vi "LTESaveDataReal1.vi"(7 "Boolean":bool, 8 "error in":errorcluster, 9 "varName":string, 10 "real1":dbl[](array[numeric])=[1.0, 2.0, 3.0], 11 "Path":path=path "C:/Users/Administrator/Desktop") -> (0 "error IO":errorcluster)   [LabVIEW 2015]
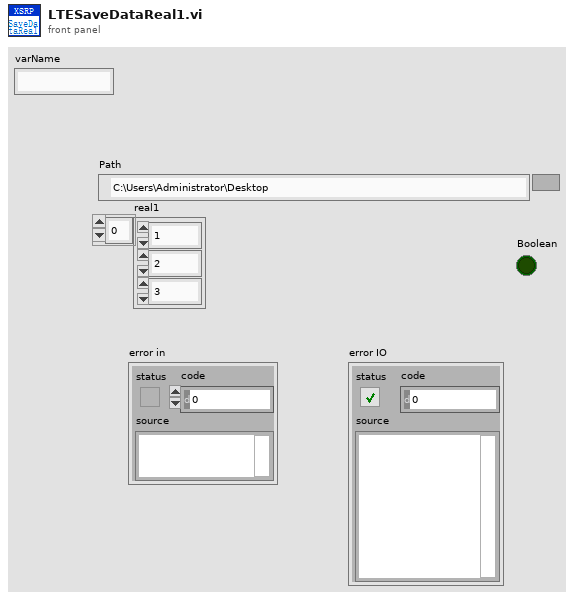
[diagram p1: front panel]
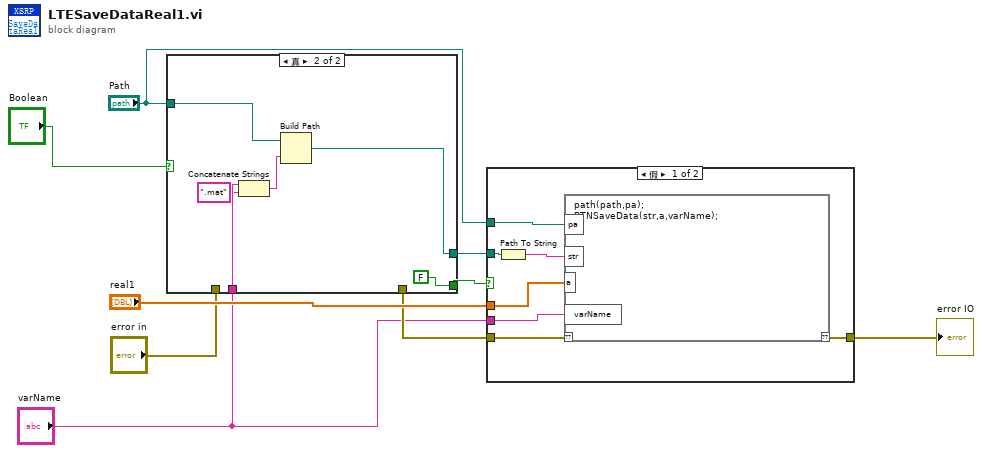
[diagram p0: block diagram]
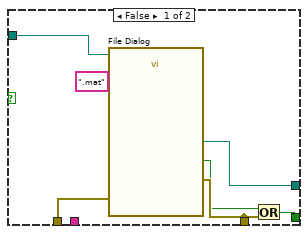
[diagram p2: hidden frame]
diagram:
  n1 = case shown="真" "Boolean" {
    tunnel: [w16 w17] -> w9
    tunnel: [w14 FALSE] -> w8
    tunnel: "Path" -> [w13 w21]
    tunnel: "error in" -> [w12 _]
    tunnel: [w11 _] -> w3
    tunnel: "varName" -> [_ w20]
    frame False {
      n2 = call "File Dialog"("start path"=w13, "error in"=w12, "pattern (all files)"=".mat") -> ("selected path"=w16:path, "cancelled"=w10:bool, "error out"=w11:errorcluster)  [unwired: 9 in, 1 out]
      n3 = Or(x=w10, y=w11) -> (x .or. y?=w14:bool)
    }
    frame True {
      n4 = Concatenate Strings(w20, ".mat" ("string")) -> (w18:string)
      n5 = Build Path(base path=w21, name or relative path=w18) -> (appended path=w17:path)
    }
  }
  n6 = case shown="假" w8 {
    tunnel: w9 -> [w29 _]
    tunnel: "Path" -> [w27 _]
    tunnel: "real1" -> [w26 _]
    tunnel: w3 -> [w25 w30]
    tunnel: [w24 w30] -> w5
    tunnel: "varName" -> [w23 _]
    frame False {
      n7 = Path To String(path=w29) -> (string=w28:string)
      n8 = script code="path(path,pa);\nBTNSaveData(str,a,varName);"("??"=w25, "pa"=w27, "a"=w26, "str"=w28, "varName"=w23) -> ("??"=w24:errorcluster)
    }
    frame True {
    }
  }
  "error IO" <- w5
